vi "Should Show Waterfall Window.vi"(10 "Data Valid":bool, 11 "Data in":T1={"First Time"=FALSE, "Show Waterfall Button Clicked"=FALSE, "Data to Process"=0.0, "Slice"=0.0, "window"=1, "averaging parameters"={"averaging mode"=enum."No averaging", "weighting mode"=enum."Exponential", "number of averages"=10}, "Waterfall VI Ref"=refnum, "Signal"={"t0"=timestamp(0 s since 1904-01-01), "dt"=0.0, "Y"=[]}} {"averaging parameters"."number of averages" min=1; "window" items=["Rectangle"=0, "Hanning"=1, "Hamming"=2, "Blackman-Harris"=3, "Exact Blackman"=4, "Blackman"=5, "Flat Top"=6, "4 Term B-Harris "=7, "7 Term B-Harris"=8, "Low Sidelobe"=9, "Blackman Nuttall"=11, "Triangle"=30, "Bartlett-Hanning"=31, "Bohman"=32, "Parzen"=33, "Welch"=34, "Kaiser"=60, "Dolph-Chebyshev"=61, "Gaussian"=62]}) -> (2 "Show Window":bool, 3 "Data out":T1={"First Time"=FALSE, "Show Waterfall Button Clicked"=FALSE, "Data to Process"=0.0, "Slice"=0.0, "window"=1, "averaging parameters"={"averaging mode"=enum."No averaging", "weighting mode"=enum."Exponential", "number of averages"=10}, "Waterfall VI Ref"=refnum, "Signal"={"t0"=timestamp(0 s since 1904-01-01), "dt"=0.0, "Y"=[]}} {"averaging parameters"."number of averages" min=1; "window" items=["Rectangle"=0, "Hanning"=1, "Hamming"=2, "Blackman-Harris"=3, "Exact Blackman"=4, "Blackman"=5, "Flat Top"=6, "4 Term B-Harris "=7, "7 Term B-Harris"=8, "Low Sidelobe"=9, "Blackman Nuttall"=11, "Triangle"=30, "Bartlett-Hanning"=31, "Bohman"=32, "Parzen"=33, "Welch"=34, "Kaiser"=60, "Dolph-Chebyshev"=61, "Gaussian"=62]})   [LabVIEW 2024, in "Waterfall.lvlib" / "Waterfall.lvclass"]
uses:
  Waterfall.lvclass
  Waterfall Data.ctl
  <vilib>/Analysis/4window.llb/windowTd.ctl
  Waterfall.lvclass/Waterfall.ctl
  <vilib>/Analysis/NI_AALPro.lvlib
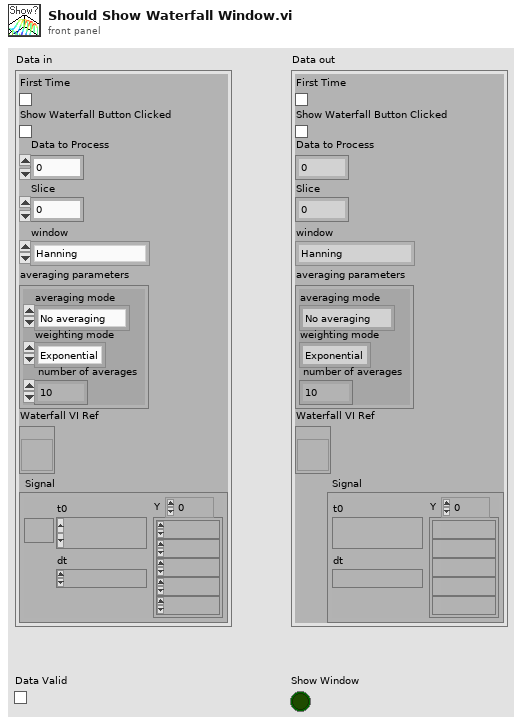
[diagram p1: front panel]
types:
  T1 = typedef "Waterfall.lvlib/Waterfall.lvclass/Waterfall Data.ctl" = cluster{"First Time":bool, "Show Waterfall Button Clicked":bool, "Data to Process":dbl, "Slice":dbl, "window":T2, "averaging parameters":cluster{"averaging mode":enum16{"No averaging", "Vector averaging", "RMS averaging", "Peak hold"}, "weighting mode":enum16{"Linear", "Exponential"}, "number of averages":u32}, "Waterfall VI Ref":refnum<vi>, "Signal":waveform(dbl)}
  T2 = typedef "NI_AALPro.lvlib/windowTd.ctl" = u32
  T3 = enum32{"Invalid", "Standard", "Closed", "Hidden", "Minimized", "Maximized"}
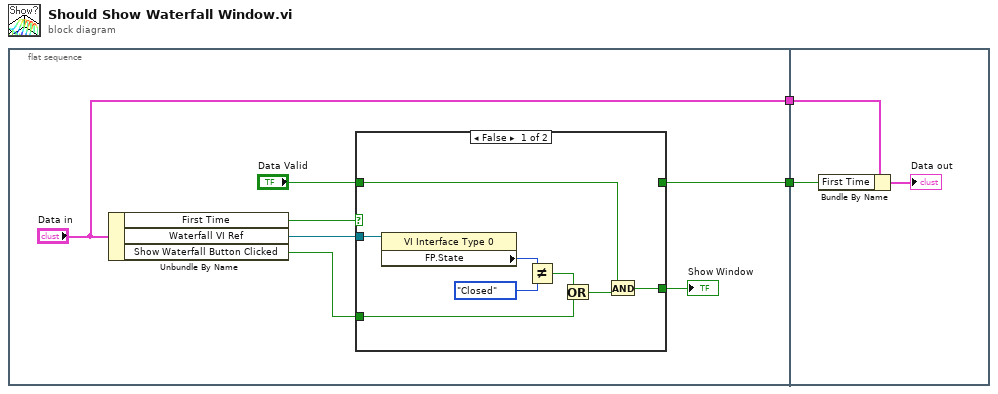
[diagram p0: block diagram]
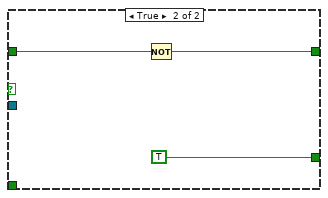
[diagram p2: hidden frame]
diagram:
  n1 = flat-sequence {
    tunnel: ["Data in"] -> w2
    tunnel: [w4] -> w1
    tunnel: w2 -> [w23]
    tunnel: w1 -> [w21]
    frame #0 {
      n2 = Unbundle By Name("Data in") -> ("First Time"=w7:bool, "Waterfall VI Ref"=w9:refnum<vi>, "Show Waterfall Button Clicked"=w8:bool)
      n3 = case shown="False" w7 {
        tunnel: w9 -> [w17 _]
        tunnel: [w10 TRUE] -> w6
        tunnel: w8 -> [w14 _]
        tunnel: [_ w19] -> w4
        tunnel: "Data Valid" -> [w11 w18]
        frame False {
          n4 = property class="VI Interface Type 0"(reference=w17) -> ("FP.State"=w16:T3)  [unwired: 1 in, 2 out]
          n5 = Not Equal?(x=w16, y=T3."Closed" ("Front Panel Window:State")) -> (x != y?=w13:bool)
          n6 = Or(x=w13, y=w14) -> (x .or. y?=w12:bool)
          n7 = And(x=w11, y=w12) -> (x .and. y?=w10:bool)
        }
        frame True {
          n8 = Not(x=w18) -> (.not. x?=w19:bool)
        }
      }
      "Show Window" <- w6
    }
    frame #1 {
      n9 = Bundle By Name(cluster=w23, "First Time"=w21) -> (→"Data out":T1)
    }
  }
